vi "morse_code_decoder.vi"() -> ()   [LabVIEW 2024]
uses:
  <vilib>/Instr/_visa.llb/VISA Configure Serial Port (Instr).vi
panel:
  out "Message":string
  out "data queue":refnum<queue>
  in  "Receiving device":refnum<visa-resource-name>
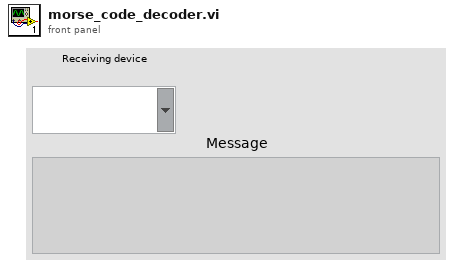
[diagram p1: front panel]
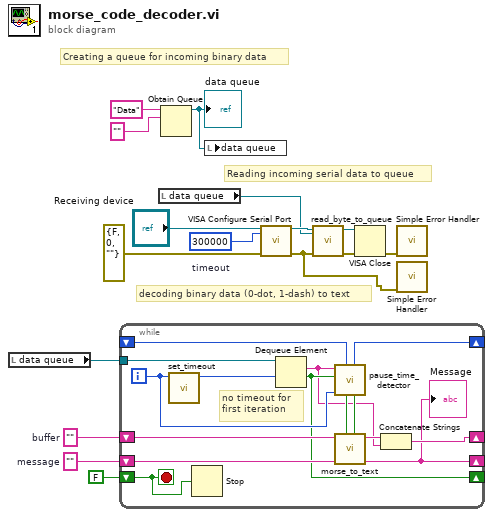
[diagram p0: block diagram]
diagram:
  w4 = ""  # buffer
  w2 = ""  # message
  w13 = u32 300000  # timeout
  # "decoding binary data (0-dot, 1-dash) to text"
  # "Reading incoming serial data to queue"
  # "Creating a queue for incoming binary data"
  n1 = local read "data queue"() -> (w9:refnum<queue>)
  n2 = while {
    tunnel: w9 -> [w31]
    shift-right: [w28] -> _
    shift-left: _ -> [w27]
    shift-right: [w20] -> _
    shift-left: FALSE ("timed out?") -> [w17]
    shift-right: [w29] -> _
    shift-left: w4 -> [w22]
    shift-right: [w18] -> _
    shift-left: w2 -> [w21]
    i -> [w23]
    stop <- w17 stop-if-true
    # "no timeout for \nfirst iteration"
    n3 = call "set_timeout.vi"("iteration count"=w23) -> ("timout value"=w30:i32)  [unwired: 10 in]
    n4 = Stop(stop? (T)=w17) -> ()
    n5 = Dequeue Element(queue=w31, timeout in ms (-1)=w30) -> (element=w19:string, timed out?=w20:bool)  [unwired: 1 in, 2 out]
    n6 = call "pause_time_detector.vi"("timestamp in"=w27, "iteration count"=w23, "end of message"=w20, "incoming character"=w19) -> ("next word"=w25:bool, "timestamp out"=w28:u32, "next letter"=w26:bool)  [unwired: 5 in]
    n7 = call "morse_to_text.vi"("next word"=w25, "next letter"=w26, "message in"=w21, "buffer in"=w22) -> ("message out"=w18:string, "buffer out"=w24:string)  [unwired: 6 in]
    "Message" <- w18
    n8 = Concatenate Strings(w24, w19) -> (w29:string)
  }
  n9 = local read "data queue"() -> (w3:refnum<queue>)
  n10 = Obtain Queue(name (unnamed)="Data", element data type="" ("name (unnamed)")) -> (queue out=w10:refnum<queue>)  [unwired: 3 in, 2 out]
  "data queue" <- w10
  n11 = local write "data queue"(w10) -> ()
  n12 = call-poly "VISA Configure Serial Port"("VISA resource name"="Receiving device", "timeout (10sec)"=w13, "error in (no error)"=errorcluster {"status"=FALSE, "code"=0, "source"=""}) -> ("VISA resource name out"=w7:refnum<visa-resource-name>, "error out"=w1:errorcluster)  [unwired: 11 in]
  n13 = call "read_byte_to_queue.vi"("Queue in"=w3, "error in (no error)"=w1, "VISA resource name in"=w7) -> ("error out"=w5:errorcluster, "VISA Refnum out"=w6:refnum<visa-resource-name>)  [unwired: 7 in]
  n14 = VISA Close(VISA resource name=w6, error in (no error)=w5) -> (error out=w15:errorcluster)
  n15 = call <vilib>:"Simple Error Handler.vi"("error in (no error)"=w15) -> ()  [unwired: 4 in, 5 out]
  n16 = call <vilib>:"Simple Error Handler.vi"("error in (no error)"=w1) -> ()  [unwired: 4 in, 5 out]
